vi "Write to table tag (SubVI).vi"(0 "alarm?":bool, 1 "Sensor Name":string, 2 "table value":refnum<vi>, 3 "Sensor Value":dbl, 5 "error in (no error)":errorcluster) -> (8 "error IO":errorcluster)   [LabVIEW 2017]
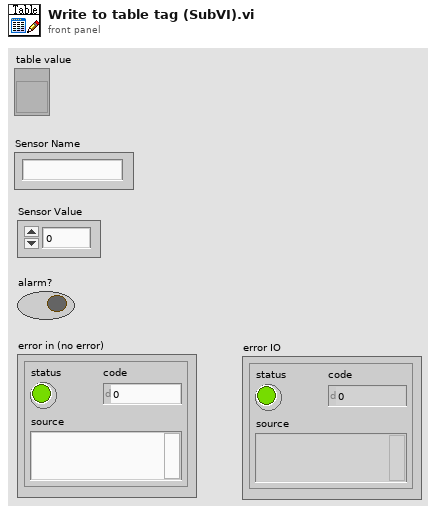
[diagram p1: front panel]
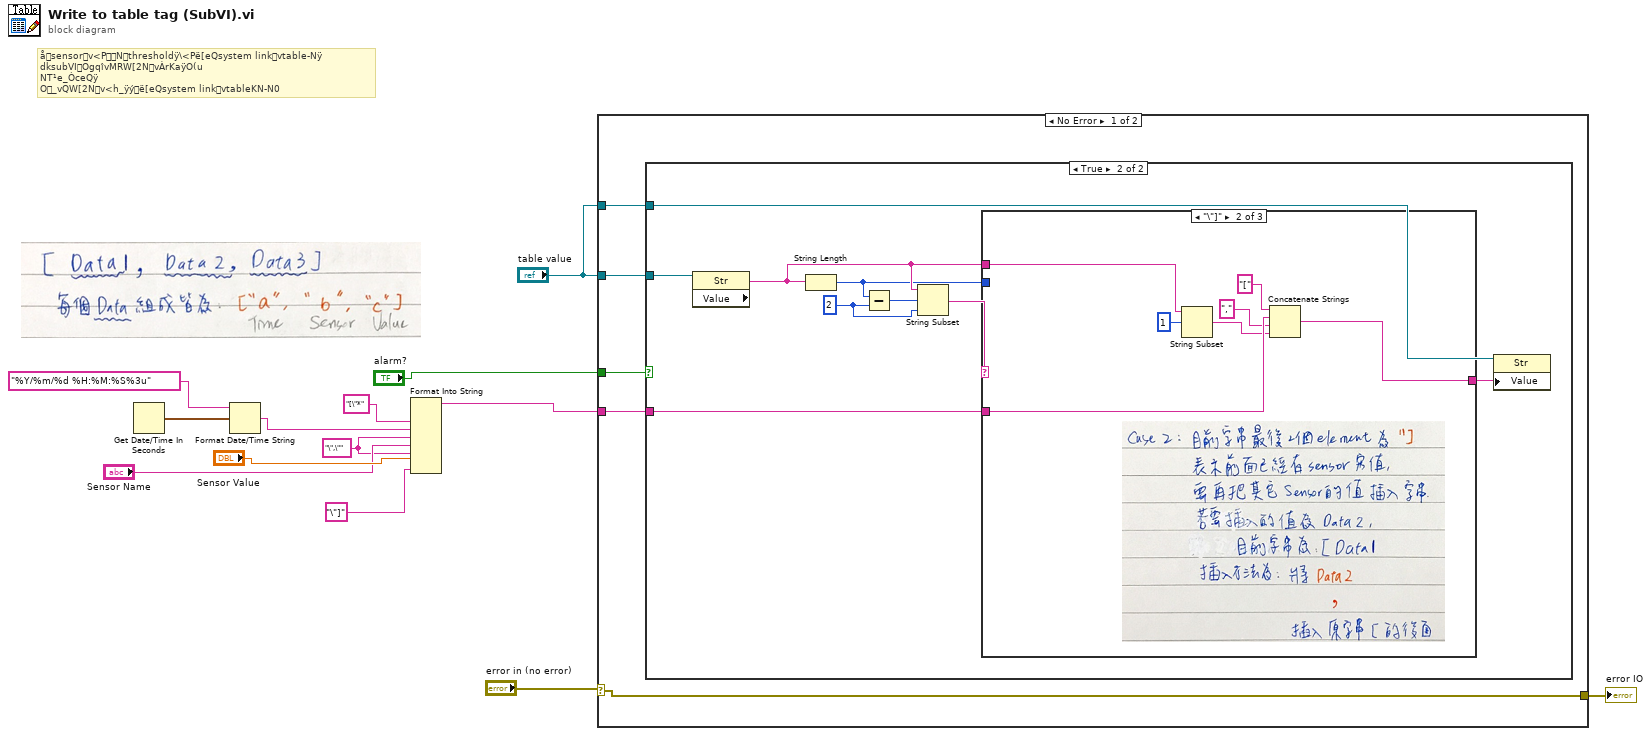
[diagram p0: block diagram]
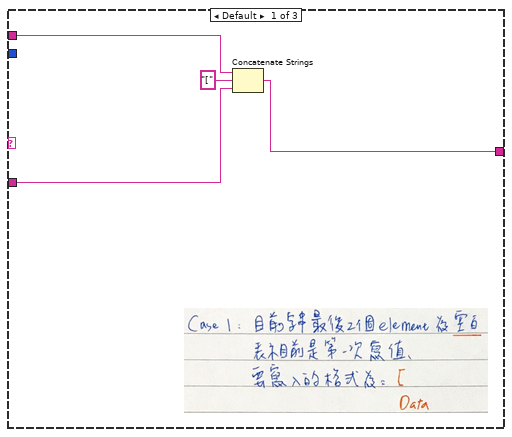
[diagram p3: hidden frame]
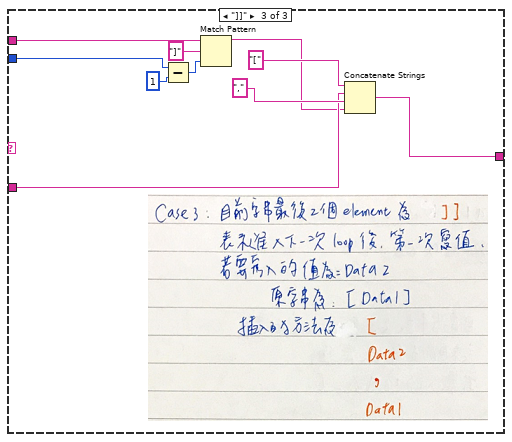
[diagram p4: hidden frame]
diagram:
  w7 = "\",\""
  # "åsensorv<PNthresholdÿ\\<Pë[eQsystem linkvtable-Nÿ\ndksubVIOgqîvMRW[2NvÀrKaÿO(u\nNT¹e_ÒceQÿ\nO_vQW[2Nv<h_ÿýë[eQsystem linkvtableKN-N0"
  n1 = Get Date/Time In Seconds() -> (seconds since 1Jan1904=w2:timestamp)
  n2 = Format Date/Time String(time format string (%c)="%Y/%m/%d %H:%M:%S%3u", seconds (now)=w2) -> (date/time string=w1:string)  [unwired: 1 in]
  n3 = Format Into String("[\"*", w1, w7, "Sensor Name", w7, "Sensor Value", "\"]") -> (resulting string=w12:string)  [unwired: 3 in, 1 out]
  n4 = case shown="No Error" "error in (no error)" {
    selector: "error in (no error)" -> [w16 w49]
    tunnel: "alarm?" -> [w18 _]
    tunnel: w12 -> [w17 _]
    tunnel: [w16 w49] -> w4
    tunnel: "table value" -> [w15 _]
    tunnel: "table value" -> [w14 _]
    frame No Error {
      n5 = case shown="True" w18 {
        tunnel: w17 -> [_ w24]
        tunnel: w15 -> [_ w20]
        tunnel: w14 -> [_ w19]
        frame False {
        }
        frame True {
          w26 = 2 ("y")
          n6 = property class="Str"(reference=w20) -> ("Value"=w22:string)  [unwired: 1 in, 2 out]
          n7 = String Length(string=w22) -> (length=w21:i32)
          n8 = Subtract(x=w21, y=w26) -> (x-y=w27:i32)
          n9 = String Subset(string=w22, offset (0)=w27, length (rest)=w26) -> (substring=w25:string)
          n10 = case shown="\"\\\"]\"" w25 {
            tunnel: w24 -> [w30 w36 w46]
            tunnel: [w28 w33 w45] -> w23
            tunnel: w22 -> [w29 w38 w40]
            tunnel: w21 -> [_ _ w43]
            frame Default {
              n11 = Concatenate Strings(w29, "[" ("string"), w30) -> (w28:string)
            }
            frame "\"]" {
              n12 = String Subset(string=w38, offset (0)=1) -> (substring=w34:string)  [unwired: 1 in]
              n13 = Concatenate Strings("[" ("string"), w36, "," ("string"), w34) -> (w33:string)
            }
            frame "]]" {
              n14 = Subtract(x=w43, y=1) -> (x-y=w41:i32)
              n15 = Match Pattern(string=w40, regular expression="]", offset (0)=w41) -> (before substring=w39:string)  [unwired: 3 out]
              n16 = Concatenate Strings("[" ("string"), w46, "," ("string"), w39) -> (w45:string)
            }
          }
          n17 = property class="Str"(reference=w19, "Value"=w23) -> ()  [unwired: 1 in, 2 out]
        }
      }
    }
    frame Error {
    }
  }
  "error IO" <- w4
